vi "Configure Modulation(BPSK).vi"(0 "VISA resource name":refnum<visa-resource-name>, 1 "Enable BPSK Modulation (F: Disable)":bool, 5 "Channel (1: Channel 1)":i32(ring)=1 items=["Channel 1"=1, "Channel 2"=2], 7 "BPSK Source (2: PN15)":i32(ring)=2 items=["01", "10", "PN15", "PN21"], 11 "error in (no error)":errorcluster, 12 "Phase (180 Degree)":dbl=180.0, 13 "BPSK Rate (100 Hz)":dbl=100.0) -> (4 "VISA resource name out":refnum<visa-resource-name>, 15 "error out":errorcluster)   [LabVIEW 2012, in "RIGOL DG4000 Series.lvlib"]
doc: "Configures BPSK (Binary Phase Shift Keying) modulation."
uses:
  <instrlib>/RIGOL DG4000 Series/RIGOL DG4000 Series.lvlib
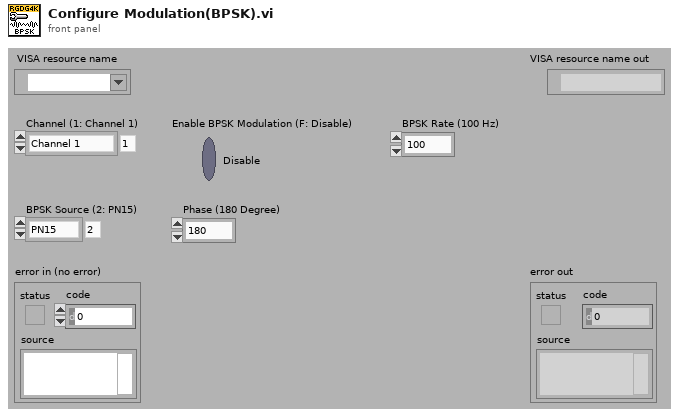
[diagram p1: front panel]
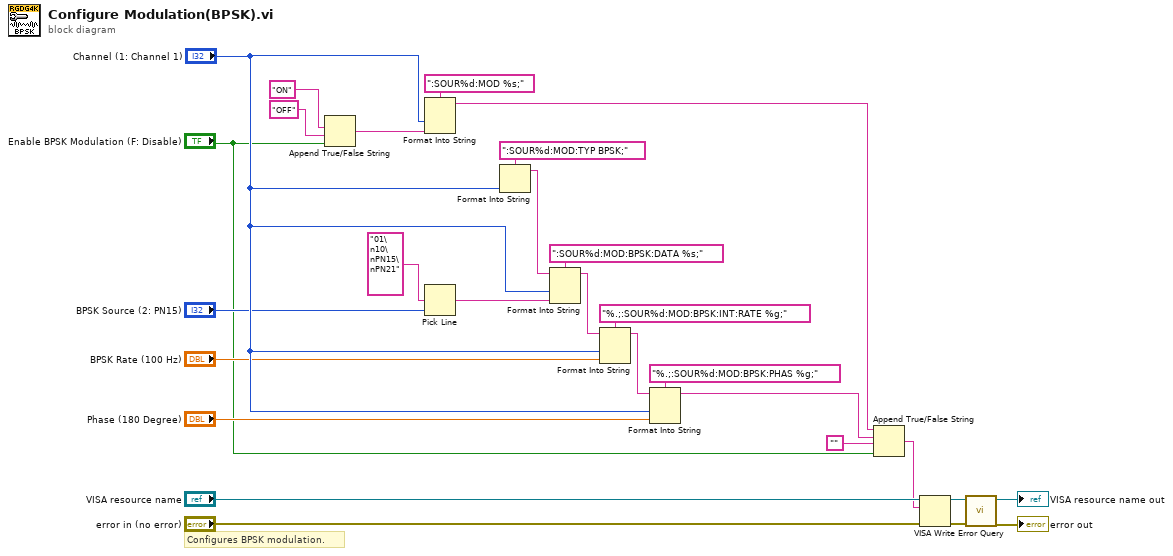
[diagram p0: block diagram]
diagram:
  # "Configures BPSK modulation."
  n1 = Append True/False String(1:"Enable BPSK Modulation (F: Disable)", 2:"OFF", 3:"ON") -> (0:w24:string)  [unwired: 1 out]
  n2 = Format Into String(format string=":SOUR%d:MOD %s;", "Channel (1: Channel 1)", w24) -> (resulting string=w2:string)  [unwired: 2 in, 1 out]
  n3 = Pick Line(multi-line string="01\n10\nPN15\nPN21", line index="BPSK Source (2: PN15)") -> (output string=w18:string)  [unwired: 1 out]
  n4 = Format Into String(format string=":SOUR%d:MOD:TYP BPSK;", "Channel (1: Channel 1)") -> (resulting string=w20:string)  [unwired: 2 in, 1 out]
  n5 = Format Into String(format string=":SOUR%d:MOD:BPSK:DATA %s;", initial string=w20, "Channel (1: Channel 1)", w18) -> (resulting string=w17:string)  [unwired: 1 in, 1 out]
  n6 = Format Into String(format string="%.;:SOUR%d:MOD:BPSK:INT:RATE %g;", initial string=w17, "Channel (1: Channel 1)", "BPSK Rate (100 Hz)") -> (resulting string=w14:string)  [unwired: 1 in, 1 out]
  n7 = Format Into String(format string="%.;:SOUR%d:MOD:BPSK:PHAS %g;", initial string=w14, "Channel (1: Channel 1)", "Phase (180 Degree)") -> (resulting string=w4:string)  [unwired: 1 in, 1 out]
  n8 = Append True/False String(1:"Enable BPSK Modulation (F: Disable)", 2:"", 3:w4, 4:w2) -> (0:w1:string)
  n9 = VISA Write(VISA resource name="VISA resource name", write buffer=w1, error in (no error)="error in (no error)") -> (VISA resource name out=w9:refnum<visa-resource-name>, error out=w8:errorcluster)  [unwired: 1 out]
  n10 = call <instrlib>:"Error Query.vi"("error in (no error)"=w8, "VISA resource name"=w9) -> ("error out"=→"error out":errorcluster, "VISA resource name out"=→"VISA resource name out":refnum<visa-resource-name>)  [unwired: 8 out]
